vi "Sort 2D Array (string).vi"(0 "Sort By":bool, 1 "Order":bool, 2 "Unsorted 2D Array":string[][](array[string])=[["", "", ""], ["", "", ""], ["", "", ""], ["", "", ""], ["", "", ""], ["", "", ""]], 3 "Column/Row to Sort By":u32, 4 "Secondary Column/Row to Sort By (-1 for None)":i32=-1) -> (5 "Sorted 2D Array":string[][](array[string]), 6 "Index Out of Range?":bool)   [LabVIEW 2025]
doc: "This VI sorts a 2D array of any size in descending or ascending order based on a column or row whose index you specify. It also allows you to use a secondary column/row, so if the main column/row has multiple elements that have the same value, it looks at the corresponding element in the secondary column/row. To use, enter an array in the Unsorted 2D Array, select whether to sort by ascending or descending order, whether to sort based on a column or row, and the primary and secondary indices of the column or row to sort by. You also can use this VI as a subVI and pass these values to it."
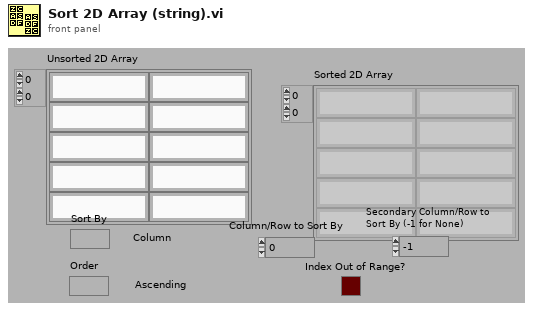
[diagram p1: front panel]
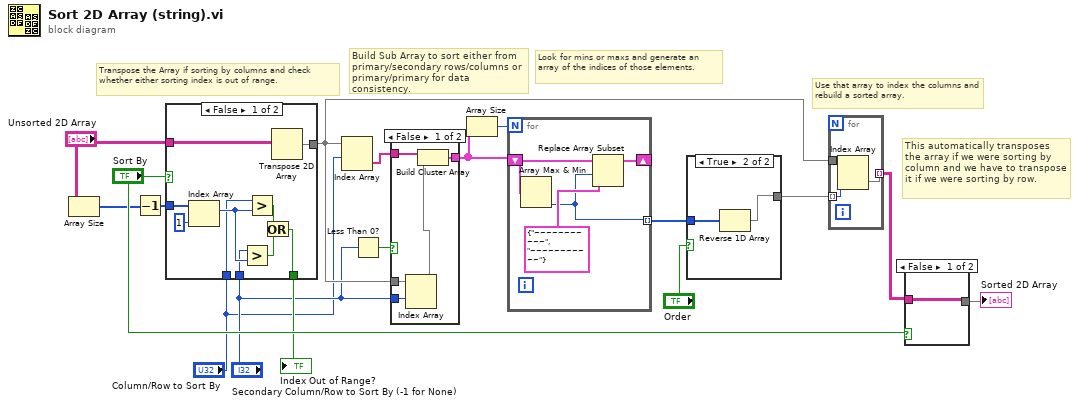
[diagram p0: block diagram]
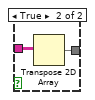
[diagram p3: hidden frame]
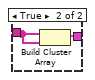
[diagram p4: hidden frame]
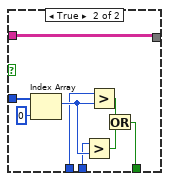
[diagram p5: hidden frame]
diagram:
  # "This automatically transposes the array if we were sorting by column and we have to transpose it if we were sorting by row."
  # "Use that array to index the columns and rebuild a sorted array."
  # "Look for mins or maxs and generate an array of the indices of those elements."
  # "Build Sub Array to sort either from primary/secondary rows/columns or primary/primary for data consistency."
  # "Transpose the Array if sorting by columns and check whether either sorting index is out of range."
  n1 = Array Size(array="Unsorted 2D Array") -> (size(s)=w8:i32[])
  n2 = Decrement(x=w8) -> (x-1=w4:i32[])
  n3 = case shown="False" "Sort By" {
    tunnel: "Unsorted 2D Array" -> [w27 w36]
    tunnel: [w26 w36] -> w13
    tunnel: w4 -> [w25 w31]
    tunnel: [w20 w30] -> w7
    tunnel: "Secondary Column/Row to Sort By (-1 for None)" -> [w18 w29]
    tunnel: "Column/Row to Sort By" -> [w19 w28]
    frame False {
      n4 = Index Array(array=w25, index=1 ("Index")) -> (element=w23:i32)
      n5 = Greater?(x=w18, y=w23) -> (0:w21:bool)
      n6 = Greater?(x=w19, y=w23) -> (0:w22:bool)
      n7 = Or(x=w22, y=w21) -> (x .or. y?=w20:bool)
      n8 = Transpose 2D Array(2D array=w27) -> (transposed array=w26:string[][])
    }
    frame True {
      n9 = Index Array(array=w31, index=0 ("Index")) -> (element=w33:i32)
      n10 = Greater?(x=w29, y=w33) -> (0:w35:bool)
      n11 = Greater?(x=w28, y=w33) -> (0:w34:bool)
      n12 = Or(x=w34, y=w35) -> (x .or. y?=w30:bool)
    }
  }
  "Index Out of Range?" <- w7
  n13 = Index Array(array=w13, index (row)="Column/Row to Sort By") -> (element=w16:string[])  [unwired: 1 in]
  n14 = Less Than 0?(x="Secondary Column/Row to Sort By (-1 for None)") -> (x < 0?=w17:bool)
  n15 = case shown="False" w17 {
    tunnel: w16 -> [w39 w42]
    tunnel: w13 -> [w41 _]
    tunnel: "Secondary Column/Row to Sort By (-1 for None)" -> [w40 _]
    tunnel: [w37 w43] -> w15
    frame False {
      n16 = Index Array(array=w41, index (row)=w40) -> (element=w38:string[])  [unwired: 1 in]
      n17 = Build Cluster Array(w39, w38) -> (w37:cluster{"String":string, "String":string}[])
    }
    frame True {
      n18 = Build Cluster Array(w42, w42) -> (w43:cluster{"String":string, "String":string}[])
    }
  }
  n19 = Array Size(array=w15) -> (size(s)=w14:i32)
  n20 = for {
    N: w14 -> [_]
    shift-right: [w46] -> _
    shift-left: w15 -> [w47]
    tunnel: [w44] -> w1 mode=indexing
    n21 = Array Max & Min(array=w47) -> (min index (indices)=w44:i32)  [unwired: 3 out]
    n22 = Replace Array Subset(array=w47, new element=cluster{"String":string, "String":string} {"String"="~~~~~~~~~~~", "String"="~~~~~~~~~~~"}, index=w44) -> (w46:cluster{"String":string, "String":string}[])
  }
  n23 = case shown="True" "Order" {
    tunnel: [w48 w49] -> w2
    tunnel: w1 -> [w48 w50]
    frame False {
    }
    frame True {
      n24 = Reverse 1D Array(array=w50) -> (reversed array=w49:i32[])
    }
  }
  n25 = for {
    tunnel: w2 -> [w53] mode=indexing
    tunnel: w13 -> [w52]
    tunnel: [w51] -> w12 mode=indexing
    n26 = Index Array(array=w52, index (col)=w53) -> (element=w51:string[])  [unwired: 1 in]
  }
  n27 = case shown="False" "Sort By" {
    tunnel: w12 -> [w54 w56]
    tunnel: [w54 w55] -> w11
    frame False {
    }
    frame True {
      n28 = Transpose 2D Array(2D array=w56) -> (transposed array=w55:string[][])
    }
  }
  "Sorted 2D Array" <- w11
